vi "rotate with temp control.vi"() -> ()   [LabVIEW 2019]
panel:
  in  "axis 2":bool=TRUE
  in  "axis 1":bool=TRUE
  in  "axis":i32
  in  "step size (deg)":dbl format="%#_13g"
  in  "final setpoint (deg)":dbl format="%#_13g"
  in  "error in":errorcluster
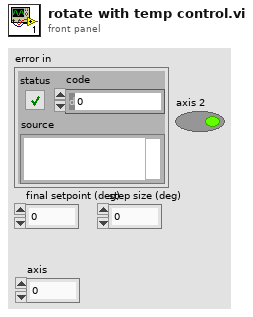
[diagram p1: front panel]
types:
  T1 = cluster{"axis 1: Amplitude [V]":dbl, "axis 2: Amplitude [V]":dbl, "axis 1: DCLevel [V]":dbl, "axis 2: DCLevel [V]":dbl, "axis 1: Frequency [Hz]":dbl, "axis 2: Frequency [Hz]":dbl, "axis 1: sp position °":dbl, "axis 2: sp position °":dbl, "axis 1: sp rot count":dbl, "axis 2: sp rot count":dbl}
  T2 = cluster{"axis 1: Absolute":bool, "axis 2: Absolute":bool, "axis 1: Stop moving":bool, "axis 2: Stop moving":bool, "axis 1: Output":bool, "axis 2: Output":bool, "set static amplitude\nwhen moving":bool}
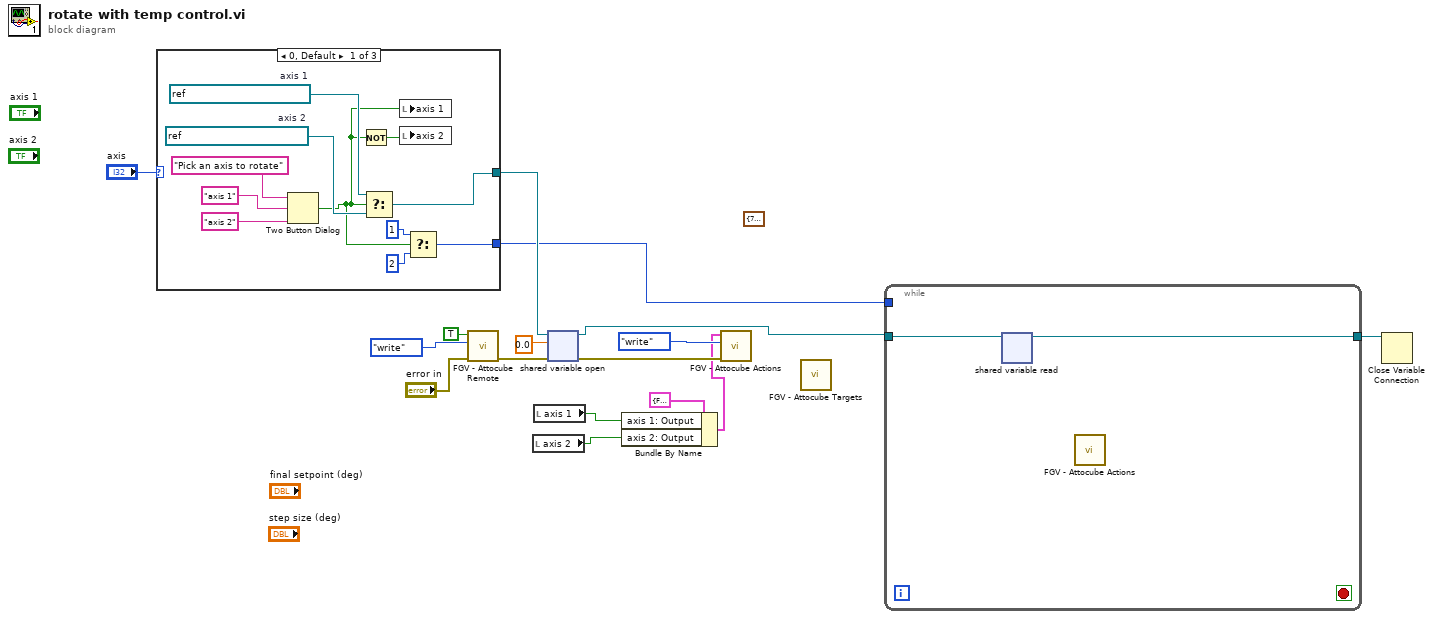
[diagram p0: block diagram]
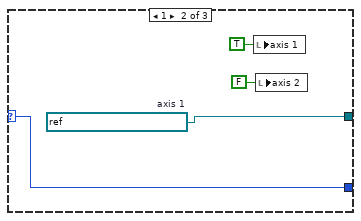
[diagram p2: hidden frame]
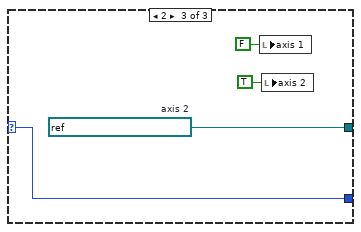
[diagram p3: hidden frame]
diagram:
  (unwired) T1 {"axis 1: Amplitude [V]"=70.0, "axis 2: Amplitude [V]"=0.0, "axis 1: DCLevel [V]"=0.0, "axis 2: DCLevel [V]"=0.0, "axis 1: Frequency [Hz]"=3500.0, "axis 2: Frequency [Hz]"=3500.0, "axis 1: sp position °"=230.0, "axis 2: sp position °"=255.0, "axis 1: sp rot count"=0.0, "axis 2: sp rot count"=0.0} ("Targets In")
  n1 = case shown="0, Default" "axis" {
    selector: "axis" -> [_ w30 w34]
    tunnel: [w22 w31 w35] -> w8
    tunnel: [w19 w30 w34] -> w6
    frame 0, Default {
      w23 = refnum<k21> "ni.var.psp://housesoftheholy/Attocube 3DR/axis 2%3A current position"  # axis 2
      w24 = refnum<k21> "ni.var.psp://housesoftheholy/Attocube 3DR/axis 1%3A current position"  # axis 1
      n2 = Two Button Dialog(message="Pick an axis to rotate", 1:"axis 2" ("F button name (\"Cancel\")"), 2:"axis 1" ("T button name (\"OK\")")) -> (T button?=w17:bool)
      n3 = Not(x=w17) -> (.not. x?=w18:bool)
      n4 = Select(t=w24, s=w17, f=w23) -> (s? t:f=w22:refnum<k21>)
      n5 = local write "axis 1"(w17) -> ()
      n6 = local write "axis 2"(w18) -> ()
      n7 = Select(t=1, s=w17, f=2) -> (s? t:f=w19:i32)
    }
    frame 1 {
      w31 = refnum<k21> "ni.var.psp://housesoftheholy/Attocube 3DR/axis 1%3A current position"  # axis 1
      n8 = local write "axis 1"(TRUE ("axis 1")) -> ()
      n9 = local write "axis 2"(FALSE ("axis 2")) -> ()
    }
    frame 2 {
      w35 = refnum<k21> "ni.var.psp://housesoftheholy/Attocube 3DR/axis 2%3A current position"  # axis 2
      n10 = local write "axis 1"(FALSE ("axis 1")) -> ()
      n11 = local write "axis 2"(TRUE ("axis 2")) -> ()
    }
  }
  n12 = call "FGV - Attocube Remote.vi"("error in"="error in", "Function"=enum16{"write", "read"}."write", "Attocube Remote"=TRUE) -> ("error out"=w13:errorcluster)  [unwired: 3 in, 1 out]
  n13 = local read "axis 2"() -> (w2:bool)
  n14 = local read "axis 1"() -> (w3:bool)
  n15 = shared-variable-open(w8, w13, 0.0 ("step size (deg) 2")) -> (w11:refnum<k21>, w7:errorcluster)
  n16 = Bundle By Name(cluster=T2 {"axis 1: Absolute"=FALSE, "axis 2: Absolute"=FALSE, "axis 1: Stop moving"=FALSE, "axis 2: Stop moving"=FALSE, "axis 1: Output"=FALSE, "axis 2: Output"=FALSE, "set static amplitude\nwhen moving"=FALSE} ("Actions IN"), "axis 1: Output"=w3, "axis 2: Output"=w2) -> (w1:T2)
  n17 = call "FGV - Attocube Actions.vi"("error in"=w7, "Function"=enum16{"write", "read"}."write", "Actions IN"=w1) -> ()  [unwired: 3 in, 2 out]
  n18 = call "FGV - Attocube Targets.vi"() -> ()  [unwired: 6 in, 2 out]
  n19 = while {
    tunnel: w11 -> [w37]
    tunnel: [w36] -> w10
    tunnel: w6 -> [_]
    stop <- _ stop-if-true
    n20 = shared-variable-read(w37) -> (w36:refnum<k21>)  [unwired: 1 in, 3 out]
    n21 = call "FGV - Attocube Actions.vi"() -> ()  [unwired: 6 in, 2 out]
  }
  n22 = Close Variable Connection(11:w10) -> ()  [unwired: 1 in, 1 out]
